vi "FlushQueue.vi"(8 "error in (no error)":errorcluster, 11 "PriorityMessageQueue in":refnum<class "PriorityMessageQueue.lvclass">) -> (0 "error out":errorcluster, 2 "Remaining Messages":refnum<class "Message.lvclass">[](array[class]), 3 "PriorityMessageQueue out":refnum<class "PriorityMessageQueue.lvclass">)   [LabVIEW 2009, in "LapDog.Messaging.v2.lvlib" / "PriorityMessageQueue.lvclass"]
doc: "<b>This class is deprecated in version 2.1 and will be removed in version 3.0</b>"
uses:
  PriorityMessageQueue.lvclass
  MessageObject/Message.lvclass
  PriorityMessageQueue.lvclass/PriorityMessageQueue.ctl
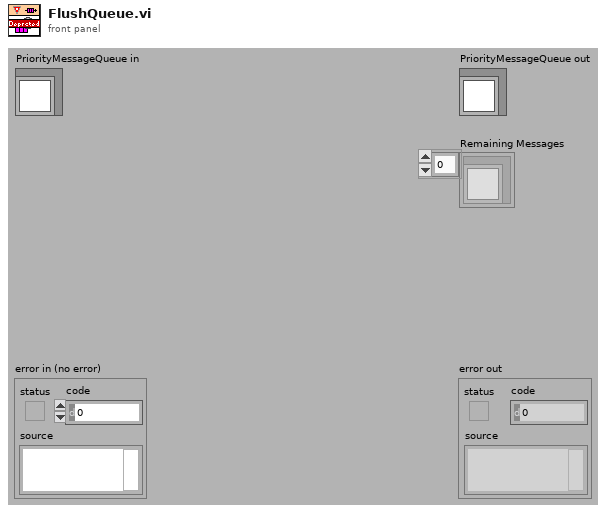
[diagram p1: front panel]
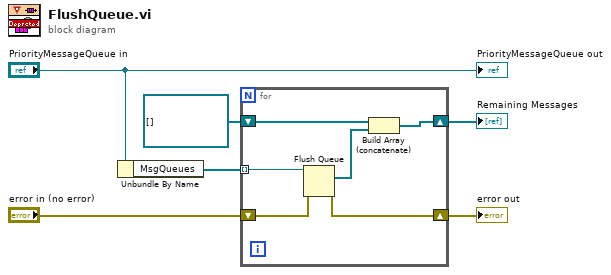
[diagram p0: block diagram]
diagram:
  n1 = Unbundle By Name("PriorityMessageQueue in") -> ("MsgQueues"=w5:refnum<queue>[])
  n2 = for {
    tunnel: w5 -> [w12] mode=indexing
    shift-right: [w10] -> w3
    shift-left: "error in (no error)" -> [w11]
    shift-right: [w8] -> w1
    shift-left: refnum<class "Message.lvclass">[] [] ("remaining elements") -> [w9]
    n3 = Flush Queue(queue=w12, error in (no error)=w11) -> (remaining elements=w7:refnum<class "Message.lvclass">[], error out=w10:errorcluster)  [unwired: 1 out]
    n4 = Build Array (concatenate)(w9, w7) -> (w8:refnum<class "Message.lvclass">[])
  }
  "error out" <- w3
  "Remaining Messages" <- w1
  "PriorityMessageQueue out" <- "PriorityMessageQueue in"
